vi "test Add Log File with Channels.vi"(8 "error in (no error)":errorcluster, 11 "TestCase in":refnum<class "Embedded Data Logger Scripting Unit Tests.lvclass">) -> (0 "error out":errorcluster, 3 "TestCase out":refnum<class "Embedded Data Logger Scripting Unit Tests.lvclass">)   [LabVIEW 2027, in "Embedded Data Logger Scripting Unit Tests.lvclass"]
uses:
  Embedded Data Logger Scripting Unit Tests.lvclass
  C:/Program Files/National Instruments/LabVIEW 2027/vi.lib/NI/VeriStand Custom Device Testing Tools/VeriStandScriptingTestCase/VeriStandScriptingTestCase.lvclass
  <vilib>/NI/VeriStand Custom Device Testing Tools/VeriStandScriptingTestCase/VeriStandScriptingTestCase.lvclass/VeriStandScriptingTestCase.ctl
  <vilib>/NI/VeriStand Custom Device Testing Tools/VeriStandScriptingTestCase/Read Target.vi
  C:/NetCoreDLL/NationalInstruments.VeriStand.SystemDefinitionAPI.dll
  NetCoreDLL/NationalInstruments.VeriStand.SystemDefinitionAPI.dll
  C:/Program Files/National Instruments/LabVIEW 2027/vi.lib/addons/_JKI Toolkits/VI Tester/TestCase.llb/TestCase.lvclass
  <vilib>/addons/_JKI Toolkits/VI Tester/TestCase.llb/TestCase.lvclass
  Embedded Data Logger Scripting.lvlib
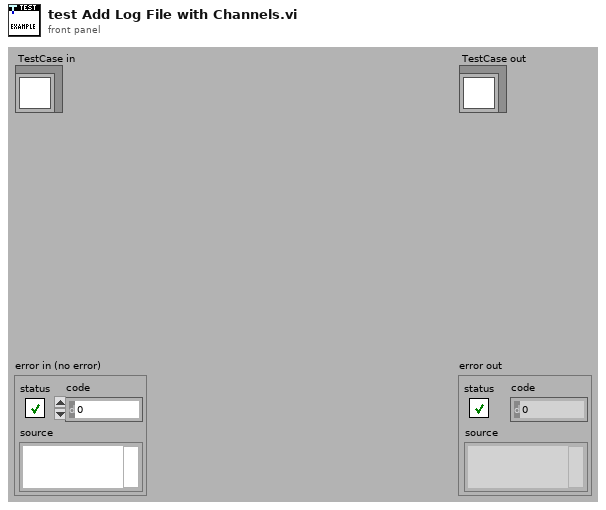
[diagram p1: front panel]
types:
  T1 = typedef "Custom Device API.lvlib/Custom Device Item Ref.ctl" = u64
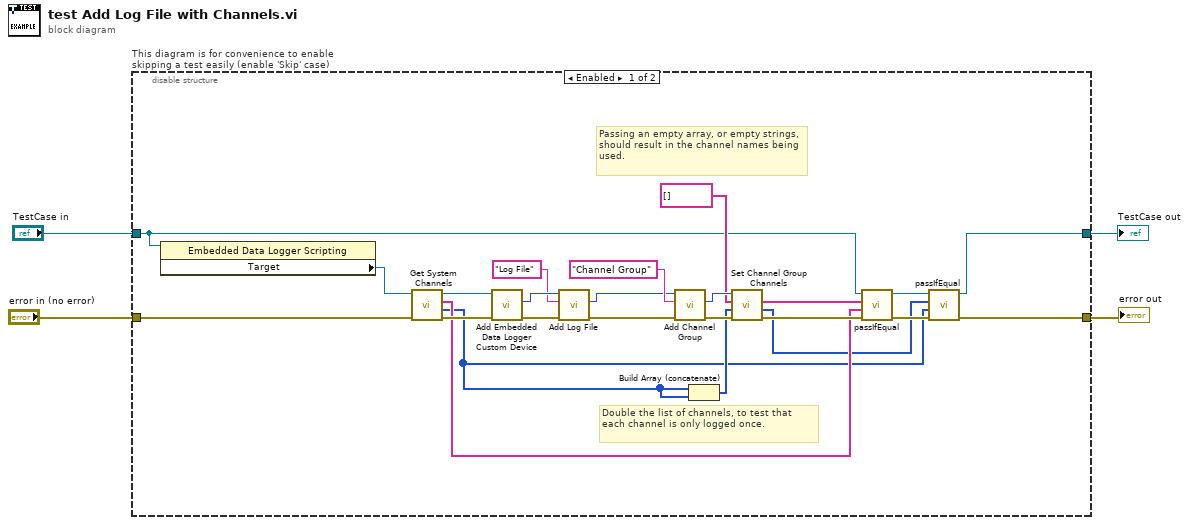
[diagram p0: block diagram]
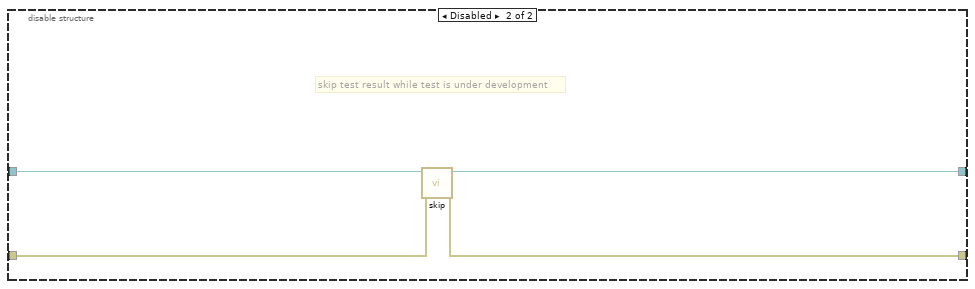
[diagram p2: hidden frame]
diagram:
  n1 = disable-structure "This diagram is for convenience to enable skipping a test easily (enable 'Skip' case)" shown="Enabled" {
    disable-tunnel: "TestCase in" -> [w14 w32]
    disable-tunnel: [w10 w30] -> w1
    disable-tunnel: [w9 w31] -> w3
    disable-tunnel: "error in (no error)" -> [w20 w29]
    frame Enabled {
      # "Passing an empty array, or empty strings, should result in the channel names being used."
      # "Double the list of channels, to test that each channel is only logged once."
      n2 = property class="Embedded Data Logger Scripting "(reference=w14) -> ("Target"=w23:refnum<k39>)  [unwired: 1 in, 2 out]
      n3 = call "Get System Channels.vi"("error in (no error)"=w20, "NationalInstruments.VeriStand.SystemDefinitionAPI.Target"=w23) -> ("error out"=w19:errorcluster, "channels"=w7:T1[], "names"=w12:string[], "NationalInstruments.VeriStand.SystemDefinitionAPI.Target"=w18:refnum<k39>)  [unwired: 6 in]
      n4 = call "Add Embedded Data Logger Custom Device.vi"("error in"=w19, "NationalInstruments.VeriStand.SystemDefinitionAPI.Target"=w18) -> ("error out"=w27:errorcluster, "embedded data logger"=w28:T1)  [unwired: 7 in, 1 out]
      n5 = call "Add Log File.vi"("error in"=w27, "log file name"="Log File", "embedded data logger in"=w28) -> ("error out"=w25:errorcluster, "log file"=w5:T1)  [unwired: 6 in, 1 out]
      n6 = call "Add Channel Group.vi"("error in"=w25, "group name"="Channel Group", "log file in"=w5) -> ("error out"=w17:errorcluster, "channel group"=w22:T1)  [unwired: 6 in, 1 out]
      n7 = Build Array (concatenate)(w7, w7) -> (w16:T1[])
      n8 = call "Set Channel Group Channels.vi"("error in"=w17, "channels"=w16, "names"=string[] [], "channel group in"=w22) -> ("error out"=w15:errorcluster, "saved channels"=w6:T1[], "saved names"=w13:string[])  [unwired: 4 in, 1 out]
      n9 = call-dynamic "passIfEqual.vi"("error in (no error)"=w15, "y"=w12, "x"=w13, "TestCase in"=w14) -> ("error out"=w8:errorcluster, "TestCase out"=w11:refnum<class "Embedded Data Logger Scripting Unit Tests.lvclass">)  [unwired: 6 in]
      n10 = call-dynamic "passIfEqual.vi"("error in (no error)"=w8, "y"=w7, "x"=w6, "TestCase in"=w11) -> ("error out"=w9:errorcluster, "TestCase out"=w10:refnum<class "Embedded Data Logger Scripting Unit Tests.lvclass">)  [unwired: 6 in]
    }
    frame Disabled {
      # "skip test result while test is under development"
      n11 = call <vilib>:"skip.vi"("error in (no error)"=w29, "TestCase in"=w32) -> ("error out"=w31:errorcluster, "TestCase out"=w30:refnum<class "Embedded Data Logger Scripting Unit Tests.lvclass">)  [unwired: 8 in]
    }
  }
  "error out" <- w3
  "TestCase out" <- w1
